vi "stitch_constant.vi"(8 "Splice params":dbl[][](array[numeric]), 9 "Const params":dbl[][](array[numeric]), 10 "Splice count":i32, 11 "X":dbl[](array[numeric])) -> (2 "Const":dbl[](array[numeric]))   [LabVIEW 2019]
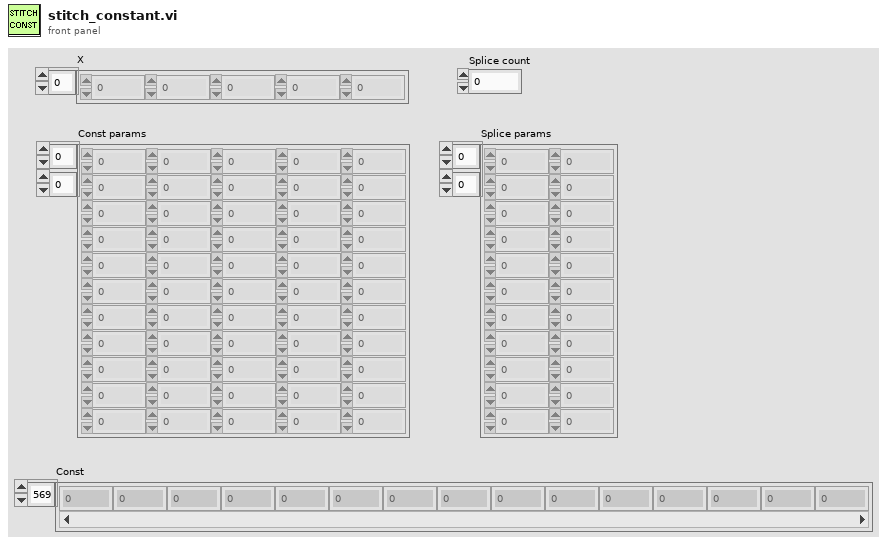
[diagram p1: front panel]
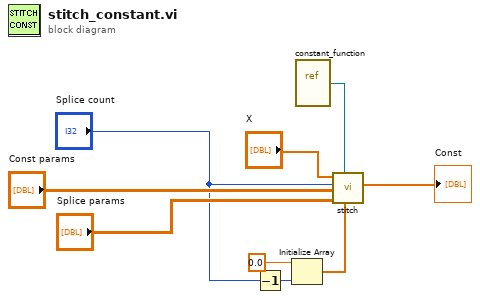
[diagram p0: block diagram]
diagram:
  n1 = Decrement(x="Splice count") -> (x-1=w4:i32)
  n2 = Initialize Array(0.0, w4) -> (w1:dbl[])
  n3 = vi-ref "constant_function.vi"() -> (w7:refnum<vi>)
  n4 = call "stitch.vi"("offsets"=w1, "f(x,a)"=w7, "splice params"="Splice params", "a"="Const params", "splice count"="Splice count", "X"="X") -> ("f(X, a)"=→"Const":dbl[])  [unwired: 5 in]
